vi "多颜色曲线.vi"() -> ()   [LabVIEW 2013]
panel:
  in  "阙值":dbl=0.5
  in  "stop":bool
  out "随机数波形图表":cluster{dbl, dbl}(graph)
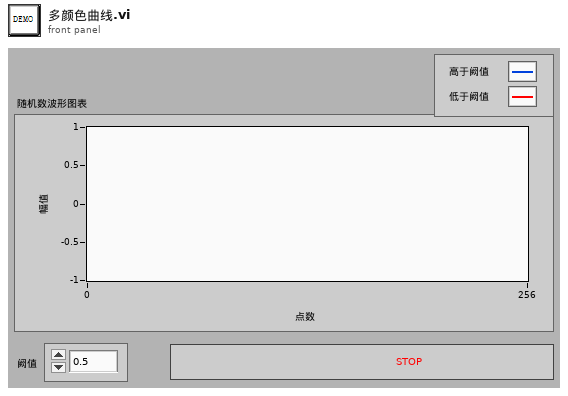
[diagram p1: front panel]
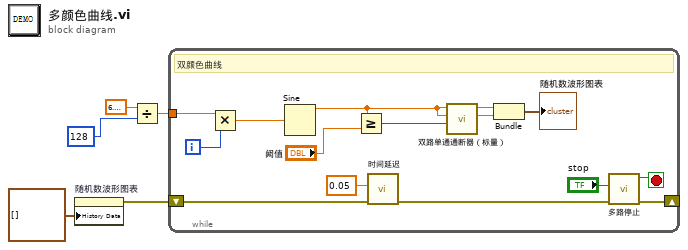
[diagram p0: block diagram]
diagram:
  n1 = property on="随机数波形图表" class="WFChart (严格)"("History Data"=cluster{dbl, dbl}[] [] ("历史数据")) -> (error out=w5:errorcluster)  [unwired: 2 in, 1 out]
  n2 = Divide(x=6.283185307179586, y=128) -> (x/y=w2:dbl)
  n3 = while {
    shift-right: [w8] -> _
    shift-left: w5 -> [w18]
    tunnel: w2 -> [w17]
    i -> [w9]
    stop <- w6 stop-if-true
    # "双颜色曲线"
    n4 = Multiply(x=w17, y=w9) -> (x*y=w16:dbl)
    n5 = Sine(x=w16) -> (sin(x)=w11:dbl)
    n6 = Greater Or Equal?(x=w11, y="阙值") -> (x >= y?=w15:bool)
    n7 = call "时间延迟"("error in (no error)"=w18, "Delay Time (s)"=0.05) -> ("error out"=w20:errorcluster)  [unwired: 9 in]
    n8 = call-poly "双路单通通断器（标量）.vi"("X直通？"=w15, "Y_In"=w11, "X_In"=w11) -> ("Y_Out"=w13:dbl, "X_Out"=w14:dbl)  [unwired: 7 in]
    n9 = Bundle("X_Out"=w14, "Y_Out"=w13) -> (→"随机数波形图表":cluster{"X_Out":dbl, "Y_Out":dbl})  [unwired: 1 in]
    n10 = call "多路停止.vi"("error in (no error)"=w20, "停止1"="stop") -> ("error in (no error)"=w8:errorcluster, "为真停止"=w6:bool)  [unwired: 6 in, 1 out]
  }
